vi "CheckForCriminalRecord.vi"(0 "Licence":string, 3 "error in":errorcluster, 4 "Database":string[][](array[string])) -> (10 "error out":errorcluster)   [LabVIEW 2019]
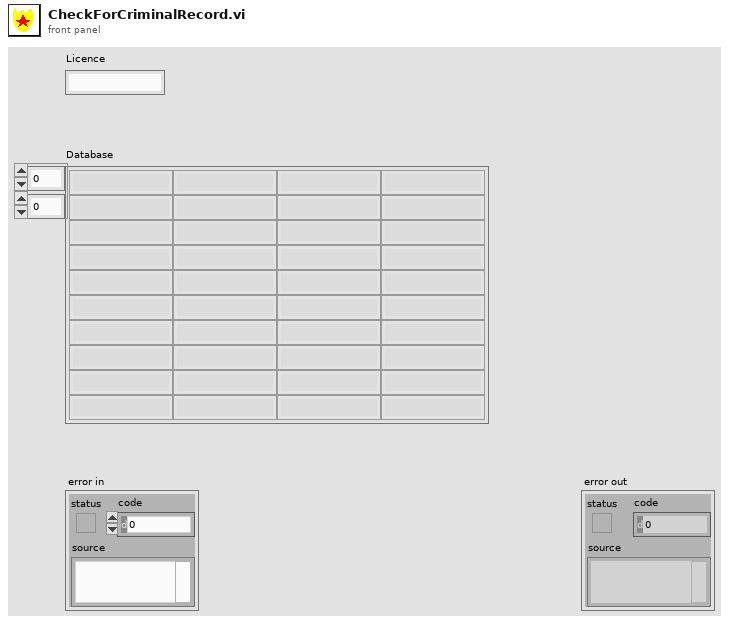
[diagram p1: front panel]
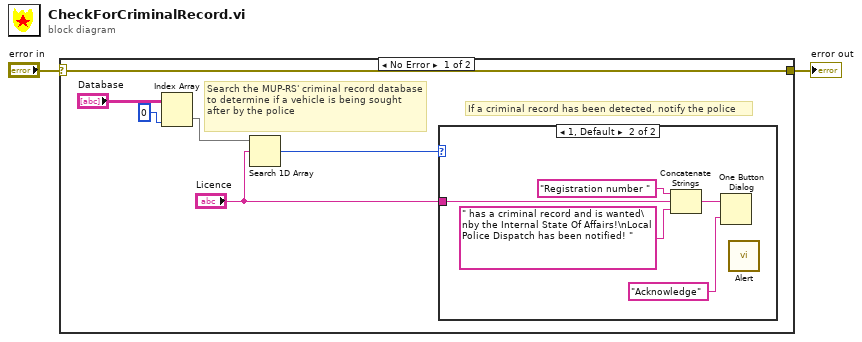
[diagram p0: block diagram]
diagram:
  n1 = case shown="No Error" "error in" {
    selector: "error in" -> [w5 w14]
    tunnel: [w5 w14] -> w1
    frame No Error {
      # "If a criminal record has been detected, notify the police"
      # "Search the MUP-RS' criminal record database to determine if a vehicle is being sought after by the police"
      n2 = Index Array(array="Database", index (col)=0 ("disabled index (col)")) -> (element=w8:string[])  [unwired: 1 in]
      n3 = Search 1D Array(1D array=w8, element="Licence") -> (index of element=w6:i32)  [unwired: 1 in]
      n4 = case shown="1, Default" w6 {
        tunnel: "Licence" -> [_ w9]
        frame -1 {
        }
        frame 1, Default {
          n5 = Concatenate Strings("Registration number " ("string"), w9, " has a criminal record and is wanted\nby the Internal State Of Affairs!\nLocal Police Dispatch has been notified! " ("string")) -> (w11:string)
          n6 = One Button Dialog(message=w11, button name ("OK")="Acknowledge") -> ()  [unwired: 1 out]
          n7 = call "Alert.vi"() -> ()  [unwired: 12 in]
        }
      }
    }
    frame Error {
    }
  }
  "error out" <- w1
